vi "PID_control.vi"() -> ()   [LabVIEW 2017]
uses:
  <instrlib>/Lake Shore Cryotronics 332/Lake Shore Cryotronics 332.lvlib
panel:
  in  "Rate(D)":dbl min=0.0 max=200.0 step=1.0
  in  "Reset (I) (0.0)":dbl min=0.0 max=1000.0 step=0.1 format="%.1f"
  in  "Gain (P)":dbl min=0.0 max=1000.0 step=0.1 format="%.1f"
  in  "Manual Output":dbl min=0.0 max=100.0 step=0.001 format="%.3f"
  in  "Heater Range ()":u16(ring) items=["Off", "Low (0.5W)", "Med (5W)", "High (50W)"]
  out "Gain (P)":dbl min=0.0 max=1000.0 step=0.1 format="%.1f"
  out "Reset (I)":dbl min=0.0 max=1000.0 step=0.1 format="%.1f"
  out "Rate (D)":dbl min=0.0 max=1000.0 step=0.1 format="%.1f"
  out "Loop 1 Heater Range":u16(ring) items=["Off", "Low (0.5W)", "Med (5W)", "High (50W)"]
  in  "Enable Powerup ()":bool
  in  "Setpoint":dbl min=-273.0 max=300000.0 step=0.0001 format="%.4f"
  in  "Control Mode":u16(ring) items=["Manual PID", "Zone", "Open Loop", "AutoTune PID", "AutoTune PI", "AutoTune P"]
  in  "VISA resource name":refnum<visa-resource-name>
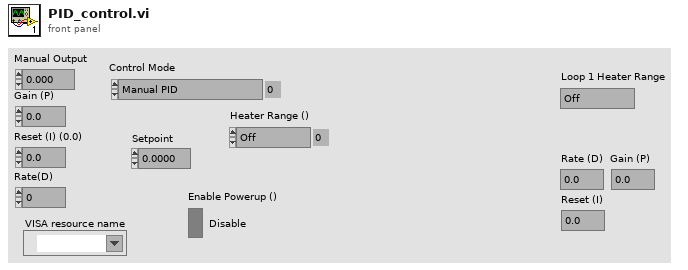
[diagram p1: front panel]
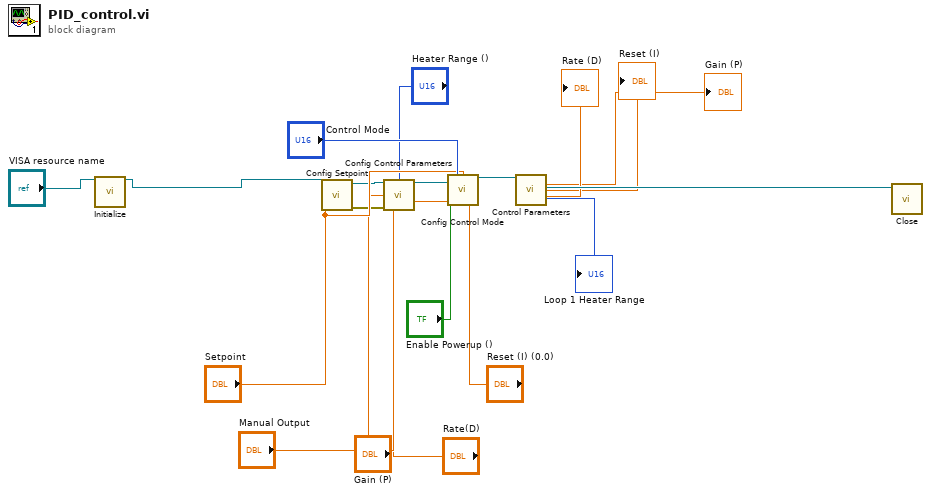
[diagram p0: block diagram]
diagram:
  n1 = call <instrlib>:"Initialize.vi"("VISA resource name"="VISA resource name") -> ("VISA resource name out"=w18:refnum<visa-resource-name>)  [unwired: 13 in, 1 out]
  n2 = call <instrlib>:"Config Setpoint.vi"("Setpoint (0.0000)"="Setpoint", "VISA resource name"=w18) -> ("error out"=w8:errorcluster, "VISA resource name out"=w9:refnum<visa-resource-name>)  [unwired: 8 in]
  n3 = call <instrlib>:"Config Control Parameters.vi"("VISA resource name"=w9, "Manual Output (0.000)"="Manual Output", "Heater Range (0: Off)"="Heater Range ()", "Gain (P) (0.0)"="Gain (P)", "Reset (I) (0.0)"="Reset (I) (0.0)", "error in (no error)"=w8, "Rate (D) (0)"="Rate(D)") -> ("VISA resource name out"=w7:refnum<visa-resource-name>)  [unwired: 7 in, 1 out]
  n4 = call <instrlib>:"Config Control Mode.vi"("VISA resource name"=w7, "Control Mode (0: Manual PID)"="Control Mode", "Setpoint Units (0: Kelvin)"="Setpoint", "Enable Powerup (F: Enable)"="Enable Powerup ()") -> ("VISA resource name out"=w1:refnum<visa-resource-name>)  [unwired: 10 in, 1 out]
  n5 = call <instrlib>:"Control Parameters.vi"("VISA resource name"=w1) -> ("VISA resource name out"=w17:refnum<visa-resource-name>, "Gain (P)"=→"Gain (P)":dbl, "Reset (I)"=→"Reset (I)":dbl, "Rate (D)"=→"Rate (D)":dbl, "Loop 1 Heater Range"=→"Loop 1 Heater Range":u16)  [unwired: 7 in, 3 out]
  n6 = call <instrlib>:"Close.vi"("VISA resource name"=w17) -> ()  [unwired: 10 in, 1 out]
